vi "Project_UI.vi"() -> ()   [LabVIEW 2019]
uses:
  <vilib>/Utility/miscctls.llb/LVPointTypeDef.ctl
  <vilib>/Utility/miscctls.llb/LVPositionTypeDef.ctl
  Class/Main Process Class/MPC_AutoPaste/Ctrl/S1 Station Input.ctl
  LLB/Message/Ctrl/MsgDataInput.ctl
  LLB/Message/Ctrl/MsgPageSelect.ctl
  LLB/Message/Ctrl/LogType.ctl
  LLB/Commonly VI/Main Glb.vi
  GLB/GLB_Project.vi
  Class/Main Process Class/Main Class.lvclass
  LLB/Commonly VI.lvlib
  LLB/Message/MsgShowAndLog.lvlib
  Class/Main Process Class/MPC_AutoPaste/Ctrl/ModbusCmd.ctl
panel:
  out "首件專案選擇":bool=TRUE
  out "dup path":path
  out "Project UI Que":refnum<queue>
  in  "Tab Control":enum32{"Page 1", "Page 2"}(tab)
  in  "Radio Buttons":enum32{"首件CHECK", "首件NO CHECK"}(radio)
  in  "Btn_Open":bool
  in  "Select Project":string caption="Project/選取專案"
  in  "Btn_Delete":bool
  in  "Btn_Copy":bool
  in  "Project List":i32(listbox) caption="專案列表/Project List"
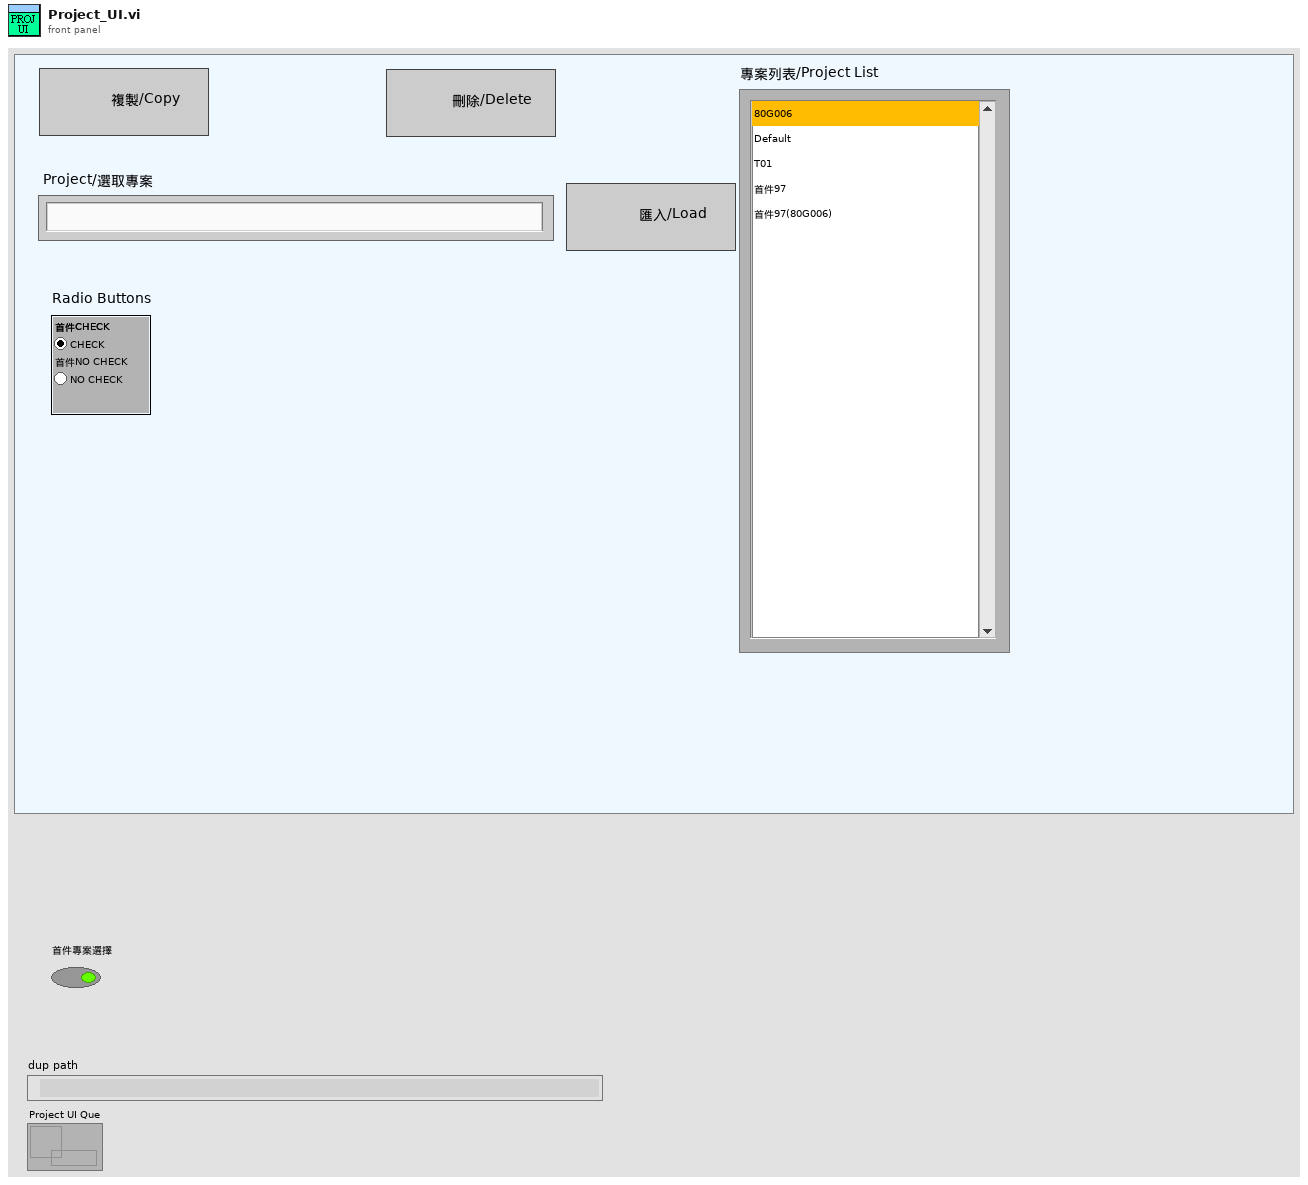
[diagram p1: front panel]
types:
  T1 = enum8{"Enabled", "Disabled", "Disabled and Grayed Out"}
  T2 = enum16{"Initial", "load", "read", "write", "write sn", "save"}
  T3 = typedef "LVPositionTypeDef.ctl" = cluster{"Left":i32, "Top":i32}
  T4 = typedef "LVPointTypeDef.ctl" = cluster{"Horizontal":i16, "Vertical":i16}
  T5 = typedef "MsgDataInput.ctl" = cluster{"MsgPageSelect":T6, "LogType":T7, "Msg":string, "Time":string}
  T6 = typedef "MsgShowAndLog.lvlib/MsgPageSelect.ctl" = enum16{"System", "Comm", "IO", "Action", "Alarm"}
  T7 = typedef "MsgShowAndLog.lvlib/LogType.ctl" = enum16{"Auto", "Manual", "Handshake", "Error"}
  T8 = enum16{"Initial", "Write", "Read", "Save", "Load", "WrteAll"}
  T9 = typedef "ModbusCmd.ctl" = enum16{"Connect", "Disconnect", "Init", "Fetch Basic Objects", "Fetch Input Refisters", "Fetch Discrete Inputs", "Set Coils", "Set Holding Registers", "Write Single Holding", "Exit"}
  T10 = typedef "S1 Station Input.ctl" = enum16{"00PLC Alive clock", "01PLC狀態(手動)", "02_備用", "03PC Recipe Change", "04PC→PLC Recipe Save", "05PC→PLC 清線", "06PC ALARM", "07PC首件模式", "08首件PASS", "09工單號碼更換", "10_S0 動作中", "11_S1條碼讀取完成", "12_備用", "13_備用", "14_備用", "15_備用", "16_備用", "17_備用", "18_備用", "19_S0載盤條碼掃描完成"}
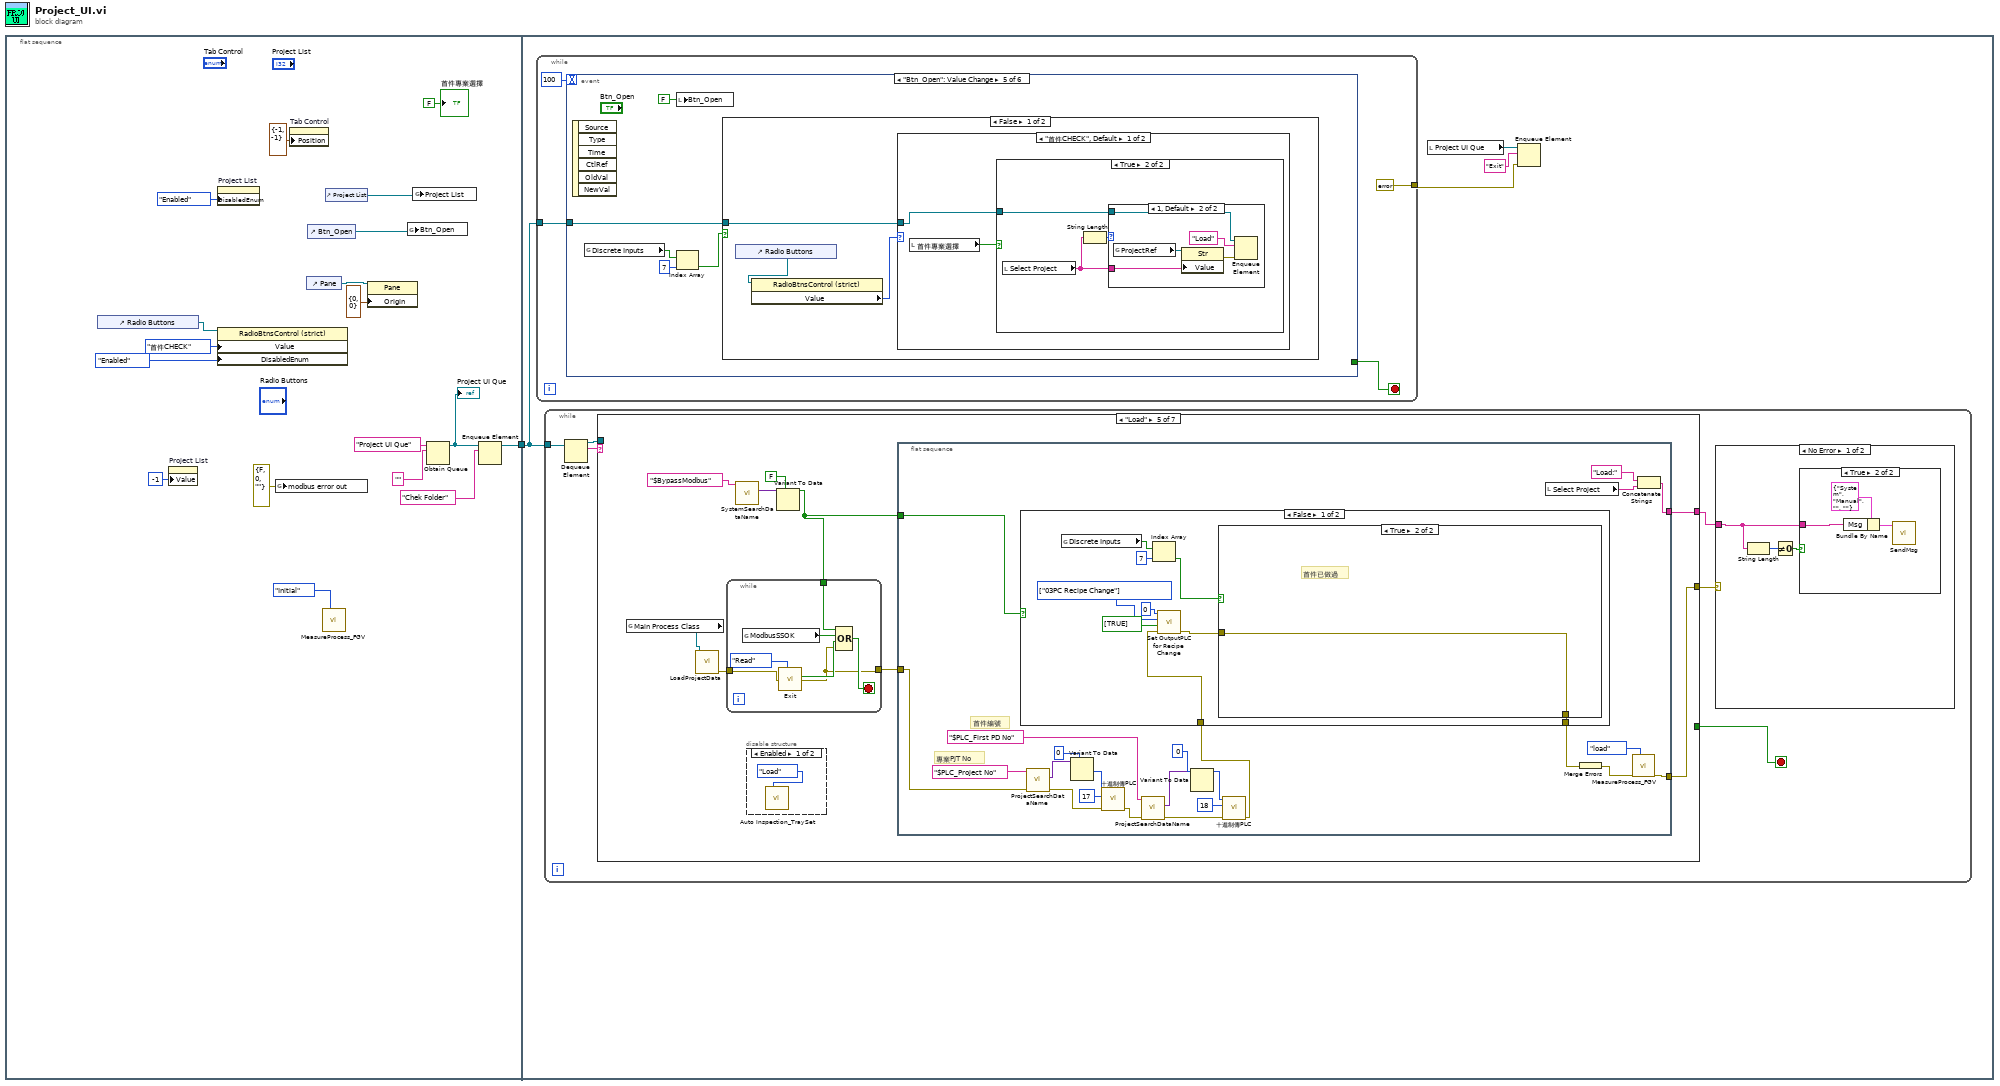
[diagram p0: block diagram]
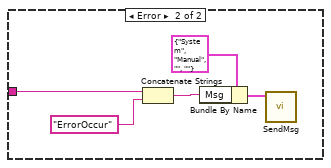
[diagram p3: hidden frame]
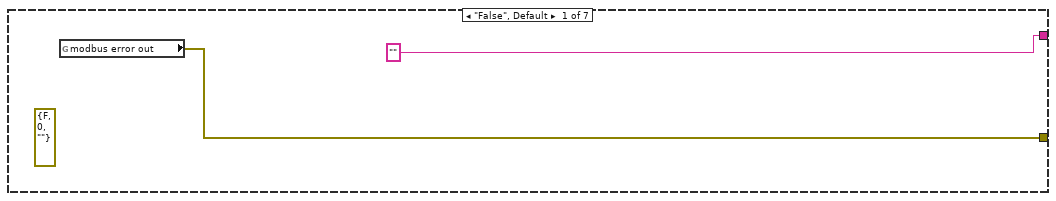
[diagram p4: hidden frame]
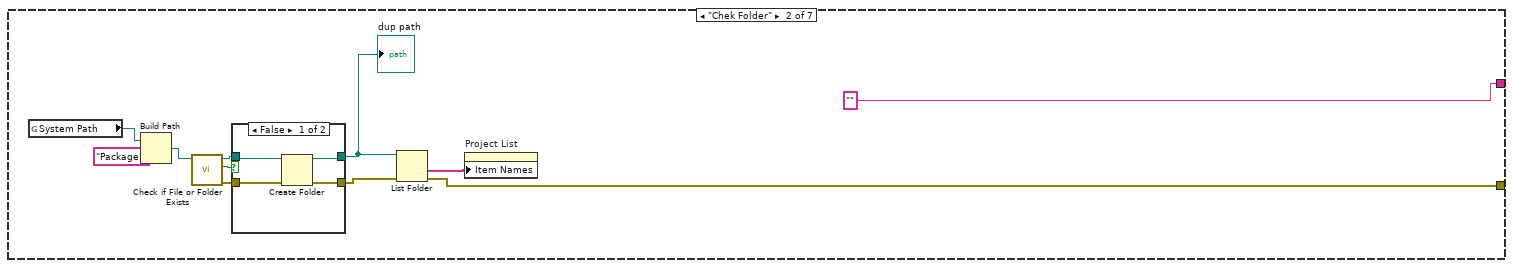
[diagram p5: hidden frame]
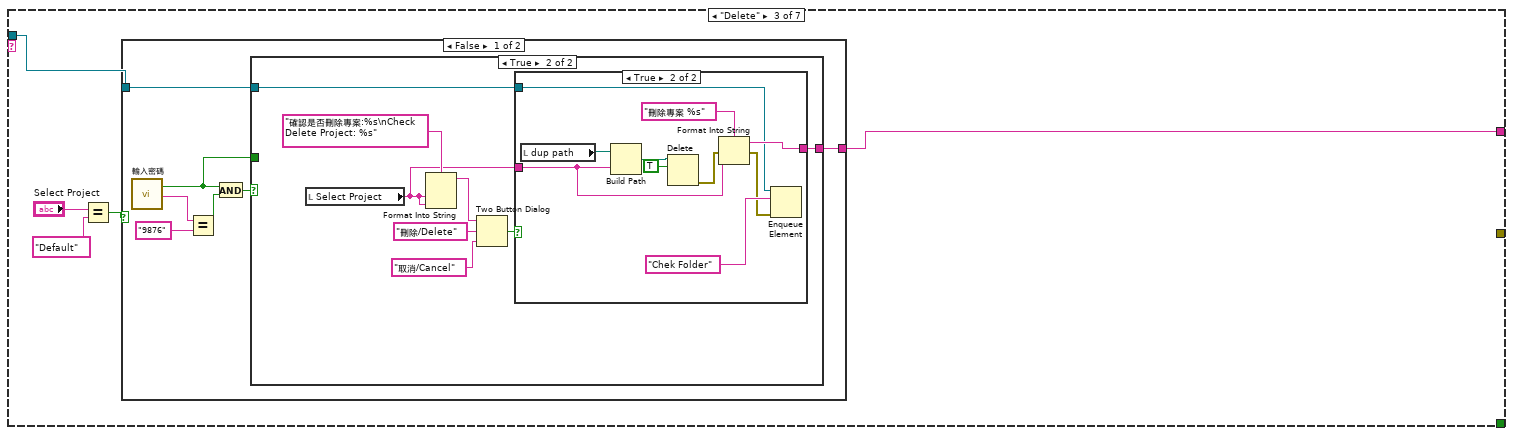
[diagram p7: hidden frame]
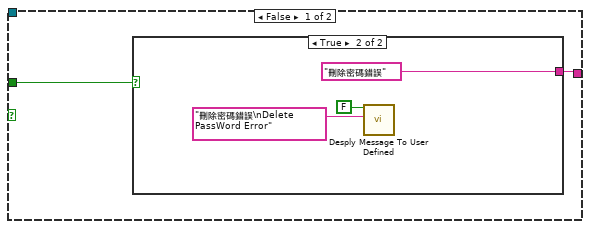
[diagram p8: hidden frame]
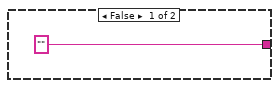
[diagram p9: hidden frame]
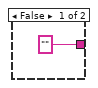
[diagram p10: hidden frame]
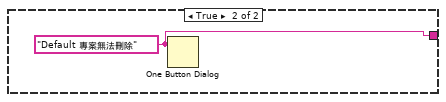
[diagram p11: hidden frame]
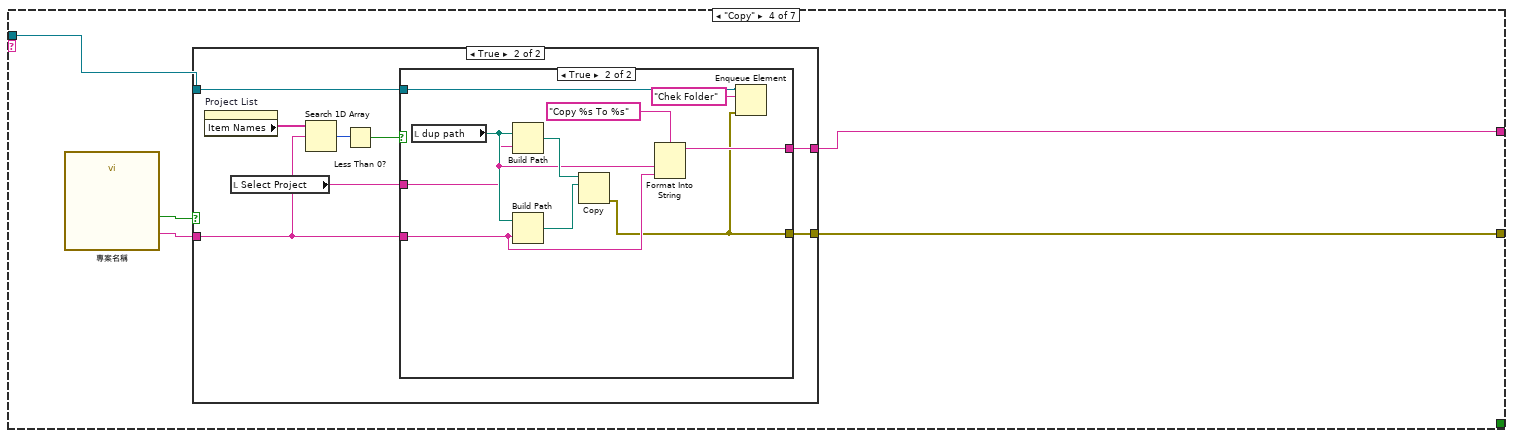
[diagram p12: hidden frame]
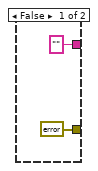
[diagram p13: hidden frame]
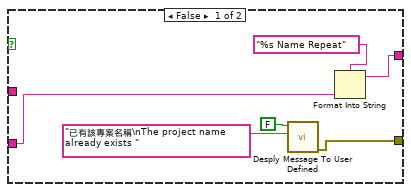
[diagram p14: hidden frame]
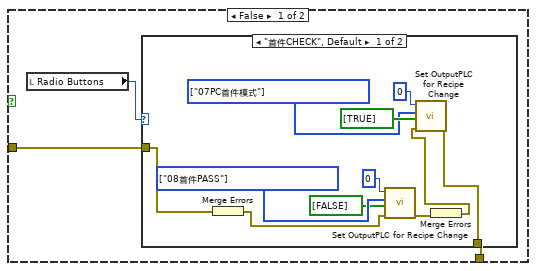
[diagram p16: hidden frame]
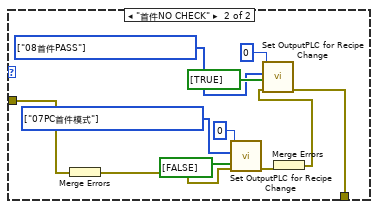
[diagram p17: hidden frame]
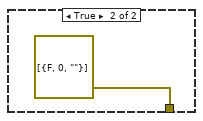
[diagram p18: hidden frame]
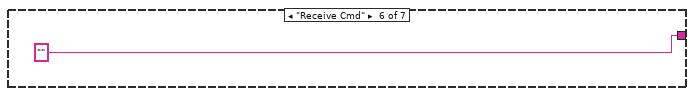
[diagram p19: hidden frame]
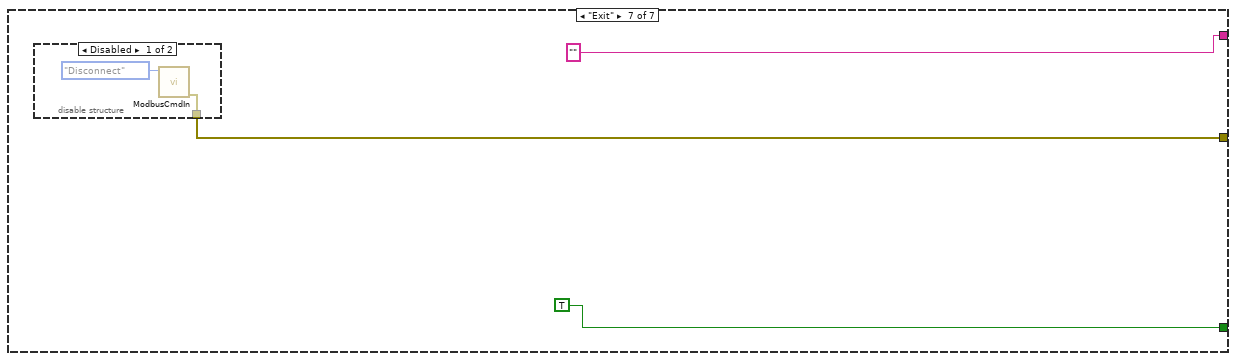
[diagram p20: hidden frame]
diagram:
  n1 = flat-sequence {
    tunnel: [w17] -> w1
    tunnel: w1 -> [w20]
    frame #0 {
      n2 = control-ref of="Radio Buttons"() -> (w4:refnum<vi>)
      n3 = property on="Project List" class="LstBox (strict)"("Value"=-1 ("Project List")) -> ()  [unwired: 2 in, 2 out]
      n4 = property on="Project List" class="LstBox (strict)"("DisabledEnum"=T1."Enabled" ("Disabled")) -> ()  [unwired: 2 in, 2 out]
      n5 = property class="RadioBtnsControl (strict)"(reference=w4, "Value"=enum32{"首件CHECK", "首件NO CHECK"}."首件CHECK", "DisabledEnum"=T1."Enabled" ("Disabled")) -> ()  [unwired: 1 in, 2 out]
      n6 = global write "Main Glb.vi" "modbus error out"(errorcluster {"status"=FALSE, "code"=0, "source"=""} ("modbus error out")) -> ()
      n7 = property on="Tab Control" class="TabCtl (strict)"("Position"=T3 {"Left"=-1, "Top"=-1}) -> ()  [unwired: 2 in, 2 out]
      n8 = control-ref of="Pane"() -> (w12:refnum<vi>)
      n9 = control-ref of="Btn_Open"() -> (w13:refnum<vi>)
      n10 = call "MeasureProcess_FGV.vi"("action"=T2."Initial") -> ()  [unwired: 10 in, 5 out]
      n11 = control-ref of="Project List"() -> (w14:refnum<vi>)
      n12 = property class="Pane"(reference=w12, "Origin"=T4 {"Horizontal"=0, "Vertical"=0}) -> ()  [unwired: 1 in, 2 out]
      n13 = global write "GLB_Project.vi" "Btn_Open"(w13) -> ()
      n14 = global write "GLB_Project.vi" "Project List"(w14) -> ()
      n15 = Obtain Queue(name (unnamed)="Project UI Que", element data type="" ("name (unnamed)")) -> (queue out=w16:refnum<queue>)  [unwired: 3 in, 2 out]
      "Project UI Que" <- w16
      n16 = Enqueue Element(queue=w16, element="Chek Folder" ("name (unnamed)")) -> (queue out=w17:refnum<queue>)  [unwired: 2 in, 2 out]
      "首件專案選擇" <- FALSE ("首件專案選擇")
    }
    frame #1 {
      n17 = while {
        tunnel: [errorcluster {"status"=FALSE, "code"=0, "source"=""} ("error constant")] -> w21
        tunnel: w20 -> [w210]
        stop <- w211 stop-if-true
        n18 = event shown="[4] \"Btn_Open\": Value Change" {
          selector: _ -> [_ _ _ _ _ _]
          dyn-events: _ -> [_ _ _ _ _ _]
          timeout: 100 -> [_ _ _ _ _ _]
          tunnel: [w215 _ _ _ _ _] -> w211
          tunnel: w210 -> [_ _ w245 w248 w253 _]
          event Timeout {
            n19 = event-data() -> ()  [unwired: 1 in, 3 out]
            n20 = call "Exit.vi"("Enum"=enum16{"Initial", "Read", "Write"}."Read") -> ("ExitOut"=w215:bool)  [unwired: 10 in]
            n21 = disable-structure shown="Disabled" {
              frame Disabled {
                n22 = global read "GLB_Project.vi" "First Run Check"() -> (w216:bool)
                n23 = case shown="False" w216 {
                  frame False {
                  }
                  frame True {
                  }
                }
              }
              frame Enabled {
              }
            }
          }
          event "Project List": Mouse Down; "Project List": Value Change {
            n24 = event-data() -> ()  [unwired: 1 in, 4 out]
            n25 = global read "Main Glb.vi" "Discrete Inputs"() -> (w219:bool[])
            n26 = Index Array(array=w219, index=7) -> (element=w217:bool)
            n27 = case shown="False" w217 {
              frame False {
                n28 = control-ref of="Radio Buttons"() -> (w221:refnum<vi>)
                n29 = property class="RadioBtnsControl (strict)"(reference=w221) -> ("Value"=w220:enum32{"首件CHECK", "首件NO CHECK"})  [unwired: 1 in, 2 out]
                n30 = case shown="\"首件CHECK\", Default" w220 {
                  frame "首件CHECK", Default {
                    w224 = "首件" ("substring (\"\")")
                    n31 = property on="Project List" class="LstBox (strict)"() -> ("Item Names"=w227:string[], "Value"=w226:i32)  [unwired: 2 in, 2 out]
                    n32 = Index Array(array=w227, index=w226) -> (element=w222:string)
                    n33 = Match Pattern(string=w222, regular expression=w224) -> (match substring=w225:string)  [unwired: 1 in, 3 out]
                    n34 = Equal?(x=w225, y=w224) -> (x = y?=w223:bool)
                    n35 = case shown="True" w223 {
                      tunnel: w222 -> [_ w231]
                      frame False {
                        n36 = disable-structure shown="Disabled" {
                          frame Disabled {
                            n37 = call "Desply Message To User Defined.vi"("Message"="請選擇首件項目") -> ()  [unwired: 9 in, 2 out]
                          }
                          frame Enabled {
                          }
                        }
                        n38 = local write "首件專案選擇"(FALSE ("首件專案選擇")) -> ()
                      }
                      frame True {
                        w230 = TRUE ("First Run Check")
                        n39 = local write "Select Project"(w231) -> ()
                        n40 = global write "GLB_Project.vi" "First Run Check"(w230) -> ()
                        n41 = local write "首件專案選擇"(w230) -> ()
                      }
                    }
                  }
                  frame "首件NO CHECK" {
                    n42 = property on="Project List" class="LstBox (strict)"() -> ("Item Names"=w234:string[], "Value"=w233:i32)  [unwired: 2 in, 2 out]
                    n43 = Index Array(array=w234, index=w233) -> (element=w232:string)
                    n44 = local write "Select Project"(w232) -> ()
                  }
                }
              }
              frame True {
                n45 = Two Button Dialog(message="已做過首件是否重做", 1:"否" ("F button name (\"Cancel\")"), 2:"是" ("T button name (\"OK\")")) -> (T button?=w235:bool)
                n46 = case shown="True" w235 {
                  frame False {
                    n47 = property on="Project List" class="LstBox (strict)"() -> ("Item Names"=w241:string[], "Value"=w240:i32)  [unwired: 2 in, 2 out]
                    n48 = Index Array(array=w241, index=w240) -> (element=w239:string)
                    n49 = local write "Select Project"(w239) -> ()
                  }
                  frame True {
                    w243 = T10[] [enum."07PC首件模式"] items=["00PLC Alive clock", "01PLC狀態(手動)", "02_備用", "03PC Recipe Change", "04PC→PLC Recipe Save", "05PC→PLC 清線", "06PC ALARM", "07PC首件模式", "08首件PASS", "09工單號碼更換", "10_S0 動作中", "11_S1條碼讀取完成", "12_備用", "13_備用", "14_備用", "15_備用", "16_備用", "17_備用", "18_備用", "19_S0載盤條碼掃描完成"]
                    n50 = call "Set OutputPLC for Recipe Change.vi"("Address In"=0, "Recipe Change"=w243, "Sat Coils"=bool[] [TRUE]) -> ()  [unwired: 7 in, 1 out]
                  }
                }
              }
            }
          }
          event "Btn_Copy": Value Change {
            n51 = event-data() -> ()  [unwired: 1 in, 6 out]
            n52 = Enqueue Element(queue=w245, element="Copy") -> ()  [unwired: 2 in, 3 out]
          }
          event "Btn_Delete": Value Change {
            n53 = event-data() -> ()  [unwired: 1 in, 6 out]
            n54 = Enqueue Element(queue=w248, element="Delete") -> ()  [unwired: 2 in, 3 out]
          }
          event "Btn_Open": Value Change {
            n55 = event-data() -> ()  [unwired: 1 in, 6 out]
            n56 = global read "Main Glb.vi" "Discrete Inputs"() -> (w251:bool[])
            n57 = local write "Btn_Open"(FALSE ("Btn_Open")) -> ()
            n58 = Index Array(array=w251, index=7) -> (element=w249:bool)
            n59 = case shown="False" w249 {
              tunnel: w253 -> [w256 w280]
              frame False {
                n60 = control-ref of="Radio Buttons"() -> (w255:refnum<vi>)
                n61 = property class="RadioBtnsControl (strict)"(reference=w255) -> ("Value"=w254:enum32{"首件CHECK", "首件NO CHECK"})  [unwired: 1 in, 2 out]
                n62 = case shown="\"首件CHECK\", Default" w254 {
                  tunnel: w256 -> [w257 w271]
                  frame "首件CHECK", Default {
                    n63 = local read "首件專案選擇"() -> (w258:bool)
                    n64 = case shown="True" w258 {
                      tunnel: w257 -> [_ w260]
                      frame False {
                        n65 = call "Desply Message To User Defined.vi"("Message"="未選取首件專案") -> ()  [unwired: 9 in, 2 out]
                      }
                      frame True {
                        n66 = local read "Select Project"() -> (w262:string)
                        n67 = String Length(string=w262) -> (length=w261:i32)
                        n68 = case shown="1, Default" w261 {
                          tunnel: w260 -> [_ w268]
                          tunnel: w262 -> [_ w265]
                          frame 0 {
                            n69 = One Button Dialog(message="請先選擇專案!!\nPlease Select Project!!") -> ()  [unwired: 1 in, 1 out]
                          }
                          frame 1, Default {
                            n70 = global read "Main Glb.vi" "ProjectRef"() -> (w266:refnum<vi>)
                            n71 = property class="Str"(reference=w266, "Value"=w265) -> (error out=w264:errorcluster)  [unwired: 1 in, 1 out]
                            n72 = Enqueue Element(queue=w268, element="Load", error in (no error)=w264) -> ()  [unwired: 1 in, 3 out]
                          }
                        }
                      }
                    }
                  }
                  frame "首件NO CHECK" {
                    n73 = local read "Select Project"() -> (w270:string)
                    n74 = String Length(string=w270) -> (length=w269:i32)
                    n75 = case shown="1, Default" w269 {
                      tunnel: w271 -> [_ w277]
                      tunnel: w270 -> [_ w274]
                      frame 0 {
                        n76 = One Button Dialog(message="請先選擇專案!!\nPlease Select Project!!") -> ()  [unwired: 1 in, 1 out]
                      }
                      frame 1, Default {
                        n77 = global read "Main Glb.vi" "ProjectRef"() -> (w275:refnum<vi>)
                        n78 = property class="Str"(reference=w275, "Value"=w274) -> (error out=w273:errorcluster)  [unwired: 1 in, 1 out]
                        n79 = Enqueue Element(queue=w277, element="Load", error in (no error)=w273) -> ()  [unwired: 1 in, 3 out]
                      }
                    }
                  }
                }
              }
              frame True {
                n80 = call "Desply Message To User Defined2.vi"("Message"="請確認首件是否完成") -> ("關閉/Close"=w278:bool)  [unwired: 9 in, 1 out]
                n81 = case shown="True" w278 {
                  tunnel: w280 -> [_ w281]
                  frame False {
                  }
                  frame True {
                    n82 = local read "Select Project"() -> (w283:string)
                    n83 = String Length(string=w283) -> (length=w282:i32)
                    n84 = case shown="1, Default" w282 {
                      tunnel: w281 -> [_ w289]
                      tunnel: w283 -> [_ w286]
                      frame 0 {
                        n85 = One Button Dialog(message="請先選擇專案!!\nPlease Select Project!!") -> ()  [unwired: 1 in, 1 out]
                      }
                      frame 1, Default {
                        n86 = global read "Main Glb.vi" "ProjectRef"() -> (w287:refnum<vi>)
                        n87 = property class="Str"(reference=w287, "Value"=w286) -> (error out=w285:errorcluster)  [unwired: 1 in, 1 out]
                        n88 = Enqueue Element(queue=w289, element="Load", error in (no error)=w285) -> ()  [unwired: 1 in, 3 out]
                      }
                    }
                  }
                }
              }
            }
          }
          event "Radio Buttons": Value Change {
            n89 = event-data() -> ()  [unwired: 1 in, 6 out]
            n90 = call "password.vi"() -> ("correct"=w290:bool)  [unwired: 11 in]
            n91 = case shown="True" w290 {
              frame False {
                n92 = control-ref of="Radio Buttons"() -> (w292:refnum<vi>)
                n93 = property class="RadioBtnsControl (strict)"(reference=w292, "Value"=enum32{"首件CHECK", "首件NO CHECK"}."首件CHECK") -> ()  [unwired: 1 in, 2 out]
              }
              frame True {
                n94 = control-ref of="Radio Buttons"() -> (w294:refnum<vi>)
                n95 = property class="RadioBtnsControl (strict)"(reference=w294) -> ("Value"=w293:enum32{"首件CHECK", "首件NO CHECK"})  [unwired: 1 in, 2 out]
                n96 = case shown="\"首件CHECK\", Default" w293 {
                  frame "首件CHECK", Default {
                    w302 = T10[] [enum."07PC首件模式"] items=["00PLC Alive clock", "01PLC狀態(手動)", "02_備用", "03PC Recipe Change", "04PC→PLC Recipe Save", "05PC→PLC 清線", "06PC ALARM", "07PC首件模式", "08首件PASS", "09工單號碼更換", "10_S0 動作中", "11_S1條碼讀取完成", "12_備用", "13_備用", "14_備用", "15_備用", "16_備用", "17_備用", "18_備用", "19_S0載盤條碼掃描完成"]
                    n97 = call "ProjectSearchDataName.vi"("element"="$PLC_First PD No") -> ("error out"=w296:errorcluster, "variant"=w297:variant)  [unwired: 7 in, 2 out]
                    n98 = Variant To Data(type=0, Variant=w297) -> (data=w301:i32)  [unwired: 1 in, 1 out]
                    n99 = call "十進制傳PLC.vi"("error in (no error)"=w296, "PLC address"=18, "Input Data"=w301) -> ("error out"=w295:errorcluster)  [unwired: 7 in, 1 out]
                    n100 = call "Set OutputPLC for Recipe Change.vi"("Address In"=0, "Recipe Change"=w302, "Sat Coils"=bool[] [TRUE], "error in (no error)"=w295) -> ()  [unwired: 6 in, 1 out]
                  }
                  frame "首件NO CHECK" {
                  }
                }
              }
            }
          }
        }
      }
      n101 = while {
        tunnel: w20 -> [w29]
        stop <- w27 stop-if-true
        n102 = Dequeue Element(queue=w29) -> (queue out=w24:refnum<queue>, element=w28:string)  [unwired: 2 in, 2 out]
        n103 = case shown="\"Load\"" w28 {
          tunnel: [_ _ _ _ _ _ TRUE] -> w27
          tunnel: [w41 w47 _ w100 w136 _ w205] -> w26
          tunnel: ["" "" w64 w99 w137 "" ("message") ""] -> w25
          tunnel: w24 -> [_ _ w63 w98 _ _ _]
          frame "False", Default {
            (unwired) errorcluster {"status"=FALSE, "code"=0, "source"=""} ("error out")
            n104 = global read "Main Glb.vi" "modbus error out"() -> (w41:errorcluster)
          }
          frame "Chek Folder" {
            n105 = global read "Main Glb.vi" "System Path"() -> (w45:path)
            n106 = Build Path(base path=w45, name or relative path="Package") -> (appended path=w44:path)
            n107 = call <vilib>:"Check if File or Folder Exists.vi"("path"=w44) -> ("error out"=w51:errorcluster, "file or folder exists?"=w53:bool, "dup path"=w52:path)  [unwired: 8 in]
            n108 = case shown="False" w53 {
              tunnel: [w56 w59] -> w50
              tunnel: w52 -> [w57 w59]
              tunnel: w51 -> [w55 w58]
              tunnel: [w54 w58] -> w48
              frame False {
                n109 = Create Folder(path (use dialog)=w57, error in=w55) -> (created path=w56:path, error out=w54:errorcluster)  [unwired: 1 in, 1 out]
              }
              frame True {
              }
            }
            "dup path" <- w50
            n110 = List Folder(path=w50, error in=w48) -> (folder names=w49:string[], error out=w47:errorcluster)  [unwired: 2 in, 2 out]
            n111 = property on="Project List" class="LstBox (strict)"("Item Names"=w49) -> ()  [unwired: 2 in, 2 out]
          }
          frame "Delete" {
            n112 = Equal?(x="Select Project", y="Default") -> (x = y?=w61:bool)
            n113 = case shown="False" w61 {
              tunnel: [w66 w97] -> w64
              tunnel: w63 -> [w65 _]
              frame False {
                n114 = call "輸入密碼"() -> ("密碼/PassWord"=w70:string, "OK"=w67:bool)  [unwired: 17 in, 1 out]
                n115 = Equal?(x=w70, y="9876") -> (x = y?=w68:bool)
                n116 = And(x=w67, y=w68) -> (x .and. y?=w71:bool)
                n117 = case shown="True" w71 {
                  tunnel: w67 -> [w73 _]
                  tunnel: [w72 w80] -> w66
                  tunnel: w65 -> [_ w78]
                  frame False {
                    n118 = case shown="True" w73 {
                      tunnel: ["" "刪除密碼錯誤"] -> w72
                      frame False {
                      }
                      frame True {
                        n119 = call "Desply Message To User Defined.vi"("Message"="刪除密碼錯誤\nDelete PassWord Error", "Show 'Cancel' Button"=FALSE) -> ()  [unwired: 8 in, 2 out]
                      }
                    }
                  }
                  frame True {
                    n120 = local read "Select Project"() -> (w79:string)
                    n121 = Format Into String(format string="確認是否刪除專案:%s\nCheck Delete Project: %s" ("Message"), w79, w79) -> (resulting string=w84:string)  [unwired: 2 in, 1 out]
                    n122 = Two Button Dialog(message=w84, 1:"取消/Cancel" ("T button name (\"OK\")"), 2:"刪除/Delete" ("T button name (\"OK\")")) -> (T button?=w81:bool)
                    n123 = case shown="True" w81 {
                      tunnel: w79 -> [_ w92]
                      tunnel: ["" w91] -> w80
                      tunnel: w78 -> [_ w87]
                      frame False {
                      }
                      frame True {
                        n124 = local read "dup path"() -> (w96:path)
                        n125 = Build Path(base path=w96, name or relative path=w92) -> (appended path=w95:path)
                        n126 = Delete(path (use dialog)=w95, entire hierarchy (F)=TRUE) -> (error out=w90:errorcluster)  [unwired: 3 in, 2 out]
                        n127 = Format Into String(format string="刪除專案 %s", error in=w90, w92) -> (resulting string=w91:string, error out=w88:errorcluster)  [unwired: 1 in]
                        n128 = Enqueue Element(queue=w87, element="Chek Folder" ("name (unnamed)"), error in (no error)=w88) -> ()  [unwired: 1 in, 3 out]
                      }
                    }
                  }
                }
              }
              frame True {
                w97 = "Default 專案無法刪除" ("message")
                n129 = One Button Dialog(message=w97) -> ()  [unwired: 1 in, 1 out]
              }
            }
          }
          frame "Copy" {
            n130 = call "專案名稱"() -> ("專案名稱/Project Name"=w102:string, "新增/Add"=w101:bool)  [unwired: 17 in, 1 out]
            n131 = case shown="True" w101 {
              tunnel: w102 -> [_ w109]
              tunnel: [errorcluster {"status"=FALSE, "code"=0, "source"=""} ("error out") w108] -> w100
              tunnel: ["" w106] -> w99
              tunnel: w98 -> [_ w105]
              frame False {
              }
              frame True {
                n132 = property on="Project List" class="LstBox (strict)"() -> ("Item Names"=w112:string[])  [unwired: 2 in, 2 out]
                n133 = local read "Select Project"() -> (w107:string)
                n134 = Search 1D Array(1D array=w112, element=w109) -> (index of element=w111:i32)  [unwired: 1 in]
                n135 = Less Than 0?(x=w111) -> (x < 0?=w110:bool)
                n136 = case shown="True" w110 {
                  tunnel: w109 -> [w113 w123]
                  tunnel: [w116 w119] -> w108
                  tunnel: w107 -> [_ w124]
                  tunnel: [w115 w122] -> w106
                  tunnel: w105 -> [_ w121]
                  frame False {
                    n137 = call "Desply Message To User Defined.vi"("Message"="已有該專案名稱\nThe project name already exists ", "Show 'Cancel' Button"=FALSE) -> ("error out"=w116:errorcluster)  [unwired: 8 in, 1 out]
                    n138 = Format Into String(format string="%s Name Repeat", w113) -> (resulting string=w115:string)  [unwired: 2 in, 1 out]
                  }
                  frame True {
                    n139 = local read "dup path"() -> (w127:path)
                    n140 = Build Path(base path=w127, name or relative path=w124) -> (appended path=w128:path)
                    n141 = Build Path(base path=w127, name or relative path=w123) -> (appended path=w126:path)
                    n142 = Copy(10:w126, 11:w128) -> (0:w119:errorcluster)  [unwired: 3 in, 2 out]
                    n143 = Format Into String(format string="Copy %s To %s", w124, w123) -> (resulting string=w122:string)  [unwired: 2 in, 1 out]
                    n144 = Enqueue Element(queue=w121, element="Chek Folder", error in (no error)=w119) -> ()  [unwired: 1 in, 3 out]
                  }
                }
              }
            }
          }
          frame "Load" {
            n145 = global read "Main Glb.vi" "Main Process Class"() -> (w131:refnum<class "Main Class.lvclass">)
            n146 = call-dynamic "LoadProjectData.vi"("Main Class in"=w131) -> ("error out"=w130:errorcluster)  [unwired: 9 in, 1 out]
            n147 = call "SystemSearchDataName.vi"("element"="$BypassModbus") -> ("variant"=w132:variant)  [unwired: 8 in, 2 out]
            n148 = disable-structure shown="Enabled" {
              frame Enabled {
                n149 = call "Auto Inspection_TraySet.vi"("Action"=T8."Load") -> ()  [unwired: 9 in, 6 out]
              }
              frame Disabled {
              }
            }
            n150 = Variant To Data(type=FALSE, Variant=w132) -> (data=w129:bool)  [unwired: 1 in, 1 out]
            n151 = while {
              tunnel: w130 -> [w140]
              tunnel: [w140] -> w135
              tunnel: w129 -> [w139]
              stop <- w141 stop-if-true
              n152 = global read "Main Glb.vi" "ModbusSSOK"() -> (w143:bool)
              n153 = call "Exit.vi"("Enum"=enum16{"Initial", "Read", "Write"}."Read") -> ("ExitOut"=w142:bool)  [unwired: 10 in]
              n154 = Compound Arithmetic op=OR(w139, w143, w142, w140) -> (w141:bool)
            }
            n155 = flat-sequence {
              tunnel: [w165] -> w137
              tunnel: [w159] -> w136
              tunnel: w135 -> [w158]
              tunnel: w129 -> [w145]
              frame #0 {
                # "首件編號"
                # "專案PJT No"
                n156 = call "ProjectSearchDataName.vi"("error in (no error)"=w158, "element"="$PLC_Project No") -> ("error out"=w157:errorcluster, "variant"=w163:variant)  [unwired: 6 in, 2 out]
                n157 = Variant To Data(type=0, Variant=w163) -> (data=w156:i32)  [unwired: 1 in, 1 out]
                n158 = call "十進制傳PLC.vi"("error in (no error)"=w157, "PLC address"=17, "Input Data"=w156) -> ("error out"=w147:errorcluster)  [unwired: 7 in, 1 out]
                n159 = call "ProjectSearchDataName.vi"("error in (no error)"=w147, "element"="$PLC_First PD No") -> ("error out"=w152:errorcluster, "variant"=w148:variant)  [unwired: 6 in, 2 out]
                n160 = Variant To Data(type=0, Variant=w148) -> (data=w153:i32)  [unwired: 1 in, 1 out]
                n161 = call "十進制傳PLC.vi"("error in (no error)"=w152, "PLC address"=18, "Input Data"=w153) -> ("error out"=w146:errorcluster)  [unwired: 7 in, 1 out]
                n162 = case shown="False" w145 {
                  tunnel: [w172 errorcluster[] [{"status"=FALSE, "code"=0, "source"=""}] ("Error Out")] -> w154
                  tunnel: w146 -> [w168 _]
                  frame False {
                    w175 = T10[] [enum."03PC Recipe Change"] items=["00PLC Alive clock", "01PLC狀態(手動)", "02_備用", "03PC Recipe Change", "04PC→PLC Recipe Save", "05PC→PLC 清線", "06PC ALARM", "07PC首件模式", "08首件PASS", "09工單號碼更換", "10_S0 動作中", "11_S1條碼讀取完成", "12_備用", "13_備用", "14_備用", "15_備用", "16_備用", "17_備用", "18_備用", "19_S0載盤條碼掃描完成"]
                    n163 = global read "Main Glb.vi" "Discrete Inputs"() -> (w171:bool[])
                    n164 = Index Array(array=w171, index=7) -> (element=w169:bool)
                    n165 = call "Set OutputPLC for Recipe Change.vi"("Address In"=0, "Recipe Change"=w175, "Sat Coils"=bool[] [TRUE], "error in (no error)"=w168) -> ("Error Out"=w173:errorcluster[])  [unwired: 6 in]
                    n166 = case shown="True" w169 {
                      tunnel: w173 -> [w178 w202]
                      tunnel: [w177 w202] -> w172
                      frame False {
                        n167 = local read "Radio Buttons"() -> (w179:enum32{"首件CHECK", "首件NO CHECK"})
                        n168 = case shown="\"首件CHECK\", Default" w179 {
                          tunnel: w178 -> [w183 w198]
                          tunnel: [w187 w197] -> w177
                          frame "首件CHECK", Default {
                            w186 = T10[] [enum."08首件PASS"] items=["00PLC Alive clock", "01PLC狀態(手動)", "02_備用", "03PC Recipe Change", "04PC→PLC Recipe Save", "05PC→PLC 清線", "06PC ALARM", "07PC首件模式", "08首件PASS", "09工單號碼更換", "10_S0 動作中", "11_S1條碼讀取完成", "12_備用", "13_備用", "14_備用", "15_備用", "16_備用", "17_備用", "18_備用", "19_S0載盤條碼掃描完成"]
                            w188 = T10[] [enum."07PC首件模式"] items=["00PLC Alive clock", "01PLC狀態(手動)", "02_備用", "03PC Recipe Change", "04PC→PLC Recipe Save", "05PC→PLC 清線", "06PC ALARM", "07PC首件模式", "08首件PASS", "09工單號碼更換", "10_S0 動作中", "11_S1條碼讀取完成", "12_備用", "13_備用", "14_備用", "15_備用", "16_備用", "17_備用", "18_備用", "19_S0載盤條碼掃描完成"]
                            n169 = Merge Errors(w183) -> (w182:errorcluster)
                            n170 = call "Set OutputPLC for Recipe Change.vi"("Address In"=0, "Recipe Change"=w186, "Sat Coils"=bool[] [FALSE], "error in (no error)"=w182) -> ("Error Out"=w181:errorcluster[])  [unwired: 6 in]
                            n171 = Merge Errors(w181) -> (w180:errorcluster)
                            n172 = call "Set OutputPLC for Recipe Change.vi"("Address In"=0, "Recipe Change"=w188, "Sat Coils"=bool[] [TRUE], "error in (no error)"=w180) -> ("Error Out"=w187:errorcluster[])  [unwired: 6 in]
                          }
                          frame "首件NO CHECK" {
                            w194 = T10[] [enum."07PC首件模式"] items=["00PLC Alive clock", "01PLC狀態(手動)", "02_備用", "03PC Recipe Change", "04PC→PLC Recipe Save", "05PC→PLC 清線", "06PC ALARM", "07PC首件模式", "08首件PASS", "09工單號碼更換", "10_S0 動作中", "11_S1條碼讀取完成", "12_備用", "13_備用", "14_備用", "15_備用", "16_備用", "17_備用", "18_備用", "19_S0載盤條碼掃描完成"]
                            w199 = T10[] [enum."08首件PASS"] items=["00PLC Alive clock", "01PLC狀態(手動)", "02_備用", "03PC Recipe Change", "04PC→PLC Recipe Save", "05PC→PLC 清線", "06PC ALARM", "07PC首件模式", "08首件PASS", "09工單號碼更換", "10_S0 動作中", "11_S1條碼讀取完成", "12_備用", "13_備用", "14_備用", "15_備用", "16_備用", "17_備用", "18_備用", "19_S0載盤條碼掃描完成"]
                            n173 = Merge Errors(w198) -> (w193:errorcluster)
                            n174 = call "Set OutputPLC for Recipe Change.vi"("Address In"=0, "Recipe Change"=w194, "Sat Coils"=bool[] [FALSE], "error in (no error)"=w193) -> ("Error Out"=w192:errorcluster[])  [unwired: 6 in]
                            n175 = Merge Errors(w192) -> (w191:errorcluster)
                            n176 = call "Set OutputPLC for Recipe Change.vi"("Address In"=0, "Recipe Change"=w199, "Sat Coils"=bool[] [TRUE], "error in (no error)"=w191) -> ("Error Out"=w197:errorcluster[])  [unwired: 6 in]
                          }
                        }
                      }
                      frame True {
                        # "首件已做過"
                      }
                    }
                  }
                  frame True {
                  }
                }
                n177 = local read "Select Project"() -> (w166:string)
                n178 = Merge Errors(w154) -> (w155:errorcluster)
                n179 = call "MeasureProcess_FGV.vi"("action"=T2."load", "error in"=w155) -> ("error out"=w159:errorcluster)  [unwired: 9 in, 4 out]
                n180 = Concatenate Strings("Load:", w166) -> (w165:string)
              }
            }
          }
          frame "Receive Cmd" {
          }
          frame "Exit" {
            n181 = disable-structure shown="Disabled" {
              disable-tunnel: [w208 _] -> w205
              frame Disabled {
                n182 = call "ModbusCmdIn.vi"("Enum"=ModbusCmd."Disconnect") -> ("error out"=w208:errorcluster)  [unwired: 10 in]
              }
              frame Enabled {
              }
            }
          }
        }
        n183 = case shown="No Error" w26 {
          tunnel: w25 -> [w32 w37]
          frame No Error {
            n184 = String Length(string=w32) -> (length=w31:i32)
            n185 = Not Equal To 0?(x=w31) -> (x != 0?=w30:bool)
            n186 = case shown="True" w30 {
              tunnel: w32 -> [_ w33]
              frame False {
              }
              frame True {
                n187 = Bundle By Name(cluster=T5 {"MsgPageSelect"=enum."System", "LogType"=enum."Manual", "Msg"="", "Time"=""} ("DataIn"), "Msg"=w33) -> (w35:T5)
                n188 = call "SendMsg.vi"("DataIn"=w35) -> ()  [unwired: 10 in, 1 out]
              }
            }
          }
          frame Error {
            n189 = Concatenate Strings(w37, "ErrorOccur") -> (w38:string)
            n190 = Bundle By Name(cluster=T5 {"MsgPageSelect"=enum."System", "LogType"=enum."Manual", "Msg"="", "Time"=""} ("DataIn"), "Msg"=w38) -> (w40:T5)
            n191 = call "SendMsg.vi"("DataIn"=w40) -> ()  [unwired: 10 in, 1 out]
          }
        }
      }
      n192 = local read "Project UI Que"() -> (w23:refnum<queue>)
      n193 = Enqueue Element(queue=w23, element="Exit", error in (no error)=w21) -> ()  [unwired: 1 in, 3 out]
    }
  }
